vi "TcM08-003_RealTime.vi"(1 "Input buffer":T3="1", 3 "Invocation info":T2, 5 "error in (no error)":errorcluster, 6 "Add log to result?":bool) -> (16 "Test Data":T1 {"Numeric Measurement" format="%.2f"}, 19 "error out":errorcluster)   [LabVIEW 2020]
doc: "Test case template."
uses:
  Shared/Support_InputBuffer.ctl
  Shared/Support_InvocationInfo.ctl
  Shared/Support_TestData.ctl
panel:
  in  "Test name":string="TcM08-003 Real-Time"
  out "Test result":bool
  out "Result":string
  # "Verify that a LabVIEW application can be executed on\na real-time target."
  # "Sub test case"
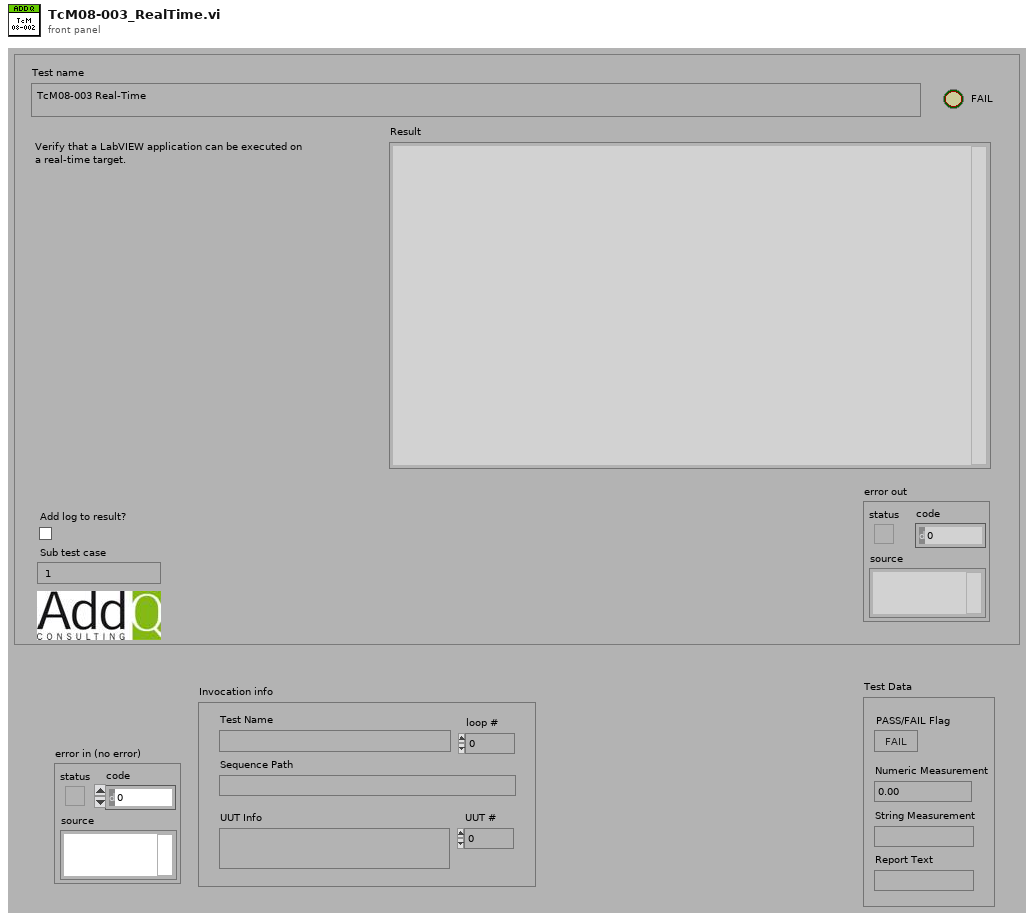
[diagram p1: front panel]
types:
  T1 = typedef "Support_TestData.ctl" = cluster{"PASS/FAIL Flag":bool, "Numeric Measurement":dbl, "String Measurement":string, "Report Text":string}
  T2 = typedef "Support_InvocationInfo.ctl" = cluster{"UUT #":i32, "loop #":i32, "UUT Info":string, "Test Name":string, "Sequence Path":path}
  T3 = typedef "Support_InputBuffer.ctl" = string
  T4 = typedef "Support_ResultType.ctl" = cluster{"Pass":bool, "Comment":string, "MeasurementValue":dbl}
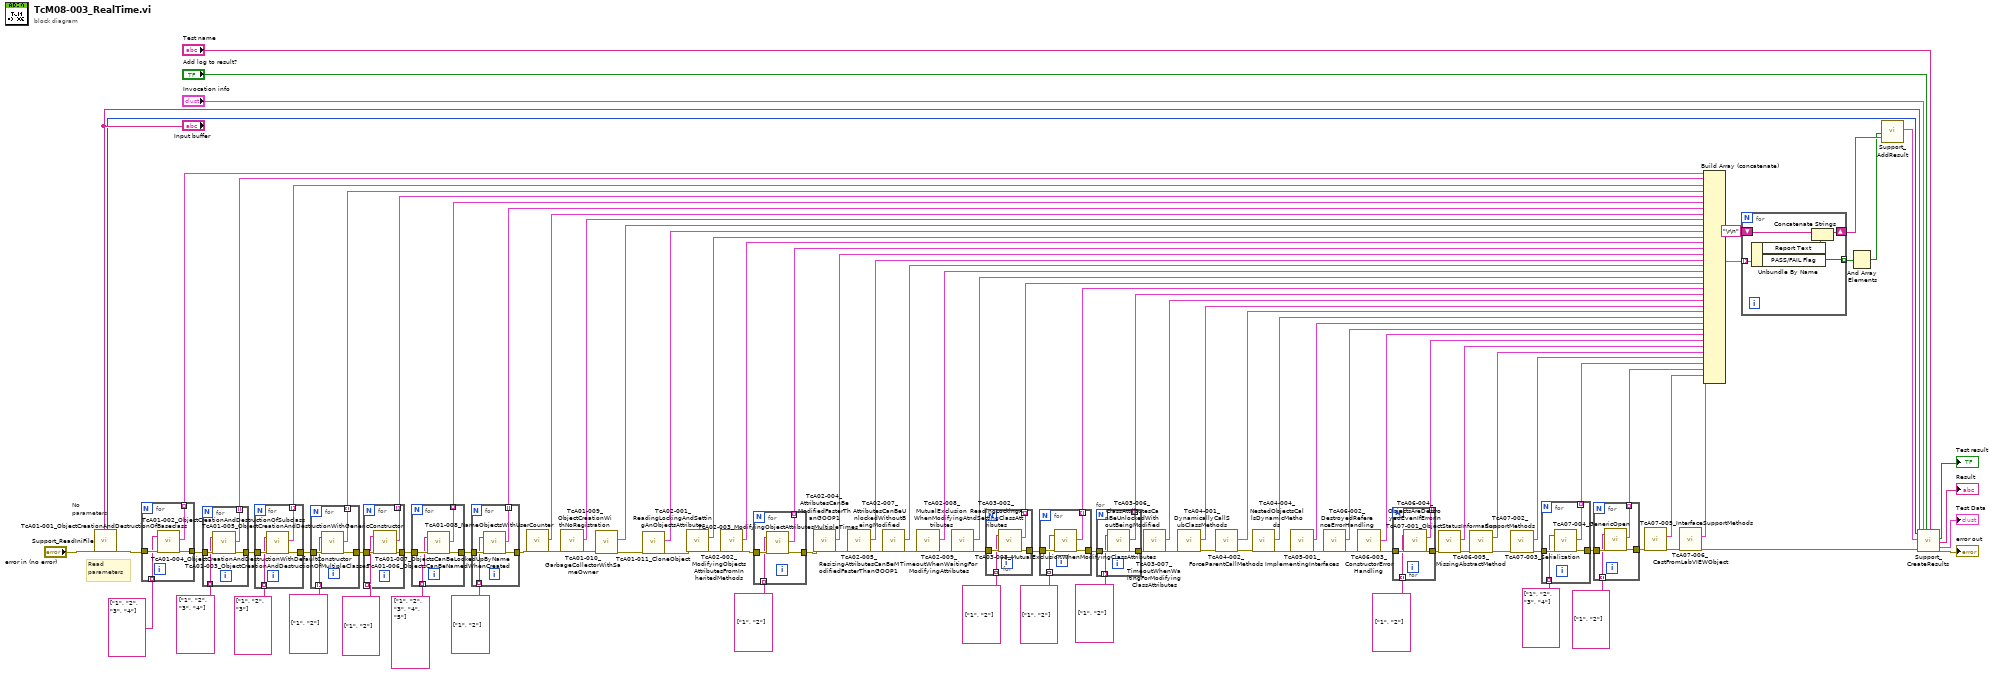
[diagram p0: block diagram]
diagram:
  # "No\nparameters"
  # "Read\nparameters"
  n1 = call "Support_ReadIniFile.vi"("error in (no error)"="error in (no error)", "Sub test case"="Input buffer") -> ("Timer start"=w95:u32, "error out"=w60:errorcluster)  [unwired: 10 in, 6 out]
  n2 = for {
    tunnel: w60 -> [w109]
    tunnel: [w108] -> w59
    tunnel: [w107] -> w58 mode=indexing
    tunnel: string[] ["1", "2", "3", "4"] -> [w106] mode=indexing
    n3 = call "TcA01-001_ObjectCreationAndDestructionOfBaseclass.vi"("Input buffer"=w106, "error in (no error)"=w109) -> ("Test Data"=w107:T1, "error out"=w108:errorcluster)  [unwired: 16 in]
  }
  n4 = for {
    tunnel: [w113] -> w94
    tunnel: [w112] -> w84 mode=indexing
    tunnel: w59 -> [w111]
    tunnel: string[] ["1", "2", "3", "4"] -> [w110] mode=indexing
    n5 = call "TcA01-002_ObjectCreationAndDestructionOfSubclass.vi"("Input buffer"=w110, "error in (no error)"=w111) -> ("Test Data"=w112:T1, "error out"=w113:errorcluster)  [unwired: 16 in]
  }
  n6 = for {
    tunnel: w94 -> [w117]
    tunnel: [w116] -> w83 mode=indexing
    tunnel: [w115] -> w47
    tunnel: string[] ["1", "2", "3"] -> [w114] mode=indexing
    n7 = call "TcA01-003_ObjectCreationAndDestructionOfMultipleClasses.vi"("Input buffer"=w114, "error in (no error)"=w117) -> ("Test Data"=w116:T1, "error out"=w115:errorcluster)  [unwired: 16 in]
  }
  n8 = for {
    tunnel: w47 -> [w121]
    tunnel: [w120] -> w46
    tunnel: [w119] -> w45 mode=indexing
    tunnel: string[] ["1", "2"] -> [w118] mode=indexing
    n9 = call "TcA01-004_ObjectCreationAndDestructionWithDefaultConstructor.vi"("Input buffer"=w118, "error in (no error)"=w121) -> ("Test Data"=w119:T1, "error out"=w120:errorcluster)  [unwired: 16 in]
  }
  n10 = for {
    tunnel: w46 -> [w125]
    tunnel: [w124] -> w44 mode=indexing
    tunnel: [w123] -> w42
    tunnel: string[] ["1", "2"] -> [w122] mode=indexing
    n11 = call "TcA01-005_ObjectCreationAndDestructionWithGenericConstructor.vi"("Input buffer"=w122, "error in (no error)"=w125) -> ("Test Data"=w124:T1, "error out"=w123:errorcluster)  [unwired: 16 in]
  }
  n12 = for {
    tunnel: [w129] -> w93
    tunnel: [w128] -> w43 mode=indexing
    tunnel: w42 -> [w127]
    tunnel: string[] ["1", "2", "3", "4", "5"] -> [w126] mode=indexing
    n13 = call "TcA01-006_ObjectsCanBeNamedWhenCreated.vi"("Input buffer"=w126, "error in (no error)"=w127) -> ("Test Data"=w128:T1, "error out"=w129:errorcluster)  [unwired: 16 in]
  }
  n14 = for {
    tunnel: w93 -> [w133]
    tunnel: [w132] -> w82 mode=indexing
    tunnel: [w131] -> w53
    tunnel: string[] ["1", "2"] -> [w130] mode=indexing
    n15 = call "TcA01-007_ObjectsCanBeLookedUpByName.vi"("Input buffer"=w130, "error in (no error)"=w133) -> ("Test Data"=w132:T1, "error out"=w131:errorcluster)  [unwired: 16 in]
  }
  n16 = call "TcA01-008_NameObjectsWithUserCounter.vi"("error in (no error)"=w53) -> ("Test Data"=w52:T1, "error out"=w35:errorcluster)  [unwired: 17 in]
  n17 = call "TcA01-009_ObjectCreationWithNoRegistration.vi"("error in (no error)"=w35) -> ("Test Data"=w34:T1, "error out"=w24:errorcluster)  [unwired: 17 in]
  n18 = call "TcA01-010_GarbageCollectorWithSameOwner.vi"("error in (no error)"=w24) -> ("Test Data"=w23:T1, "error out"=w21:errorcluster)  [unwired: 17 in]
  n19 = call "TcA01-011_CloneObject.vi"("error in (no error)"=w21) -> ("Test Data"=w19:T1, "error out"=w20:errorcluster)  [unwired: 17 in]
  n20 = call "TcA02-001_ReadingLockingAndSettingAnObjectsAttributes.vi"("error in (no error)"=w20) -> ("Test Data"=w81:T1, "error out"=w57:errorcluster)  [unwired: 17 in]
  n21 = call "TcA02-002_ModifyingObjectsAttributesFromInheritedMethods.vi"("error in (no error)"=w57) -> ("Test Data"=w55:T1, "error out"=w56:errorcluster)  [unwired: 17 in]
  n22 = for {
    tunnel: [w137] -> w92
    tunnel: [w136] -> w80 mode=indexing
    tunnel: w56 -> [w135]
    tunnel: string[] ["1", "2"] -> [w134] mode=indexing
    n23 = call "TcA02-003_ModifyingObjectAttributesMultipleTimes.vi"("Input buffer"=w134, "error in (no error)"=w135) -> ("Test Data"=w136:T1, "error out"=w137:errorcluster)  [unwired: 16 in]
  }
  n24 = call "TcA02-004_AttributesCanBeModifiedFasterThanGOOP1.vi"("error in (no error)"=w92) -> ("Test Data"=w79:T1, "error out"=w91:errorcluster)  [unwired: 17 in]
  n25 = call "TcA02-005_ResizingAttributesCanBeModifiedFasterThanGOOP1.vi"("error in (no error)"=w91) -> ("Test Data"=w78:T1, "error out"=w48:errorcluster)  [unwired: 17 in]
  n26 = call "TcA02-007_AttributesCanBeUnlockedWithoutBeingModified.vi"("error in (no error)"=w48) -> ("Test Data"=w77:T1, "error out"=w90:errorcluster)  [unwired: 17 in]
  n27 = call "TcA02-008_MutualExclusionWhenModifyingAttributes.vi"("error in (no error)"=w90) -> ("Test Data"=w76:T1, "error out"=w89:errorcluster)  [unwired: 17 in]
  n28 = call "TcA02-009_TimeoutWhenWaitingForModifyingAttributes.vi"("error in (no error)"=w89) -> ("Test Data"=w75:T1, "error out"=w49:errorcluster)  [unwired: 17 in]
  n29 = for {
    tunnel: [w141] -> w88
    tunnel: [w140] -> w74 mode=indexing
    tunnel: w49 -> [w139]
    tunnel: string[] ["1", "2"] -> [w138] mode=indexing
    n30 = call "TcA03-002_ReadingLockingAndSettingClassAttributes.vi"("Input buffer"=w138, "error in (no error)"=w139) -> ("Test Data"=w140:T1, "error out"=w141:errorcluster)  [unwired: 16 in]
  }
  n31 = for {
    tunnel: w88 -> [w145]
    tunnel: [w144] -> w73 mode=indexing
    tunnel: [w143] -> w51
    tunnel: string[] ["1", "2"] -> [w142] mode=indexing
    n32 = call "TcA03-003_MutualExclusionWhenModifyingClassAttributes.vi"("Input buffer"=w142, "error in (no error)"=w145) -> ("Test Data"=w144:T1, "error out"=w143:errorcluster)  [unwired: 16 in]
  }
  n33 = for {
    tunnel: [w149] -> w87
    tunnel: [w148] -> w72 mode=indexing
    tunnel: w51 -> [w147]
    tunnel: string[] ["1", "2"] -> [w146] mode=indexing
    n34 = call "TcA03-006_ClassAttributesCanBeUnlockedWithoutBeingModified.vi"("Input buffer"=w146, "error in (no error)"=w147) -> ("Test Data"=w148:T1, "error out"=w149:errorcluster)  [unwired: 16 in]
  }
  n35 = call "TcA03-007_TimeoutWhenWaitingForModifyingClassAttributes.vi"("error in (no error)"=w87) -> ("Test Data"=w71:T1, "error out"=w50:errorcluster)  [unwired: 17 in]
  n36 = call "TcA04-001_DynamicallyCallSubClassMethods.vi"("error in (no error)"=w50) -> ("Test Data"=w70:T1, "error out"=w3:errorcluster)  [unwired: 17 in]
  n37 = call "TcA04-002_ForceParentCallMethods.vi"("error in (no error)"=w3) -> ("Test Data"=w1:T1, "error out"=w2:errorcluster)  [unwired: 17 in]
  n38 = call "TcA04-004_NestedObjectsCallsDynamicMethods.vi"("error in (no error)"=w2) -> ("Test Data"=w69:T1, "error out"=w33:errorcluster)  [unwired: 17 in]
  n39 = call "TcA05-001_ImplementingInterfaces.vi"("error in (no error)"=w33) -> ("Test Data"=w31:T1, "error out"=w32:errorcluster)  [unwired: 17 in]
  n40 = call "TcA06-002_DestroyedReferenceErrorHandling.vi"("error in (no error)"=w32) -> ("Test Data"=w68:T1, "error out"=w86:errorcluster)  [unwired: 17 in]
  n41 = call "TcA06-003_ConstructorErrorHandling.vi"("error in (no error)"=w86) -> ("Test Data"=w67:T1, "error out"=w85:errorcluster)  [unwired: 17 in]
  n42 = for {
    tunnel: w85 -> [w153]
    tunnel: [w152] -> w66 mode=indexing
    tunnel: [w151] -> w30
    tunnel: string[] ["1", "2"] -> [w150] mode=indexing
    n43 = call "TcA06-004_ObjectsAreDestroyedEvenIfErrorIn.vi"("Input buffer"=w150, "error in (no error)"=w153) -> ("Test Data"=w152:T1, "error out"=w151:errorcluster)  [unwired: 16 in]
  }
  n44 = call "TcA06-005_MissingAbstractMethod.vi"("error in (no error)"=w30) -> ("Test Data"=w28:T1, "error out"=w29:errorcluster)  [unwired: 17 in]
  n45 = call "TcA07-001_ObjectStatusInformation.vi"("error in (no error)"=w29) -> ("Test Data"=w65:T1, "error out"=w41:errorcluster)  [unwired: 17 in]
  n46 = call "TcA07-002_SupportMethods.vi"("error in (no error)"=w41) -> ("Test Data"=w39:T1, "error out"=w40:errorcluster)  [unwired: 17 in]
  n47 = for {
    tunnel: w40 -> [w157]
    tunnel: [w156] -> w38 mode=indexing
    tunnel: [w155] -> w37
    tunnel: string[] ["1", "2", "3", "4"] -> [w154] mode=indexing
    n48 = call "TcA07-003_Serialization.vi"("Input buffer"=w154, "error in (no error)"=w157) -> ("Test Data"=w156:T1, "error out"=w155:errorcluster)  [unwired: 16 in]
  }
  n49 = for {
    tunnel: w37 -> [w161]
    tunnel: [w160] -> w36 mode=indexing
    tunnel: [w159] -> w27
    tunnel: string[] ["1", "2"] -> [w158] mode=indexing
    n50 = call "TcA07-004_GenericOpen.vi"("Input buffer"=w158, "error in (no error)"=w161) -> ("Test Data"=w160:T1, "error out"=w159:errorcluster)  [unwired: 16 in]
  }
  n51 = call "TcA07-005_InterfaceSupportMethods.vi"("error in (no error)"=w27) -> ("Test Data"=w26:T1, "error out"=w25:errorcluster)  [unwired: 17 in]
  n52 = call "TcA07-006_CastFromLabVIEWObject.vi"("error in (no error)"=w25) -> ("Test Data"=w22:T1, "error out"=w6:errorcluster)  [unwired: 17 in]
  n53 = Build Array (concatenate)(w58, w84, w83, w45, w44, w43, w82, w52, w34, w23, w19, w81, w55, w80, w79, w78, w77, w76, w75, w74, w73, w72, w71, w70, w1, w69, w31, w68, w67, w66, w28, w65, w39, w38, w36, w26, w22) -> (w64:T1[])
  n54 = for {
    tunnel: w64 -> [w166] mode=indexing
    tunnel: [w165] -> w62 mode=indexing
    shift-right: [w162] -> w63
    shift-left: "\r\n" -> [w163]
    n55 = Unbundle By Name(w166) -> ("Report Text"=w164:string, "PASS/FAIL Flag"=w165:bool)
    n56 = Concatenate Strings(w163, w164) -> (w162:string)
  }
  n57 = And Array Elements(Boolean array=w62) -> (logical AND=w61:bool)
  n58 = call "Support_AddResult.vi"("Pass"=w61, "Comment"=w63) -> ("Results out"=w98:T4[])  [unwired: 17 in]
  n59 = call "Support_CreateResults.vi"("Sub test case"="Input buffer", "Timer start"=w95, "Results"=w98, "error in (no error)"=w6, "Invocation info"="Invocation info", "Add log to result?"="Add log to result?", "Test name"="Test name") -> ("Pass/fail flag"=→"Test result":bool, "Result"=→"Result":string, "Test Data"=→"Test Data":T1, "error out"=→"error out":errorcluster)  [unwired: 9 in]
